vi "4521_Module_configure.vi"() -> ()   [LabVIEW 2010]
panel:
  in  "Port Name":string
  in  "Data Bits":u8=8 min=5 max=8 step=1
  in  "Parity type":bool
  in  "Use parity?":bool
  in  "Stop Bits":bool
  in  "Behaviour":bool
  in  "Enable Checksum?":bool
  in  "422 or 485?":bool
  in  "Append CR?":bool
  in  "485 Baud Rate (9600)":u8(ring)=3 items=["1200 bps", "2400 bps", "4800 bps", "9600 bps", "19.2 kbps", "38.4 kbps"]
  in  "Use checksum":bool
  in  "232 Baud Rate (9600)":u8(ring)=3 items=["1200 bps", "2400 bps", "4800 bps", "9600 bps", "19.2 kbps", "38.4 kbps"]
  out "Reply":string
  out "String Sent":string
  in  "New Address (NN)":u8
  in  "Old Address(AA)":u8
  # "4520 Settings"
  # "Serial Device Settings"
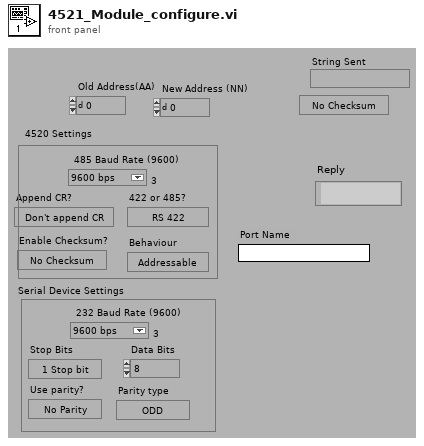
[diagram p1: front panel]
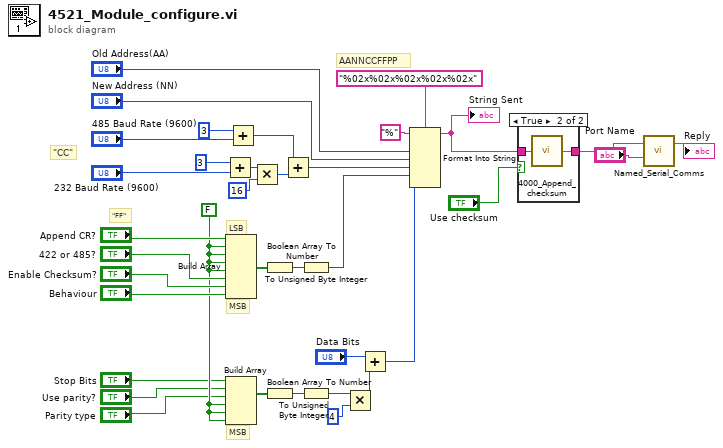
[diagram p0: block diagram]
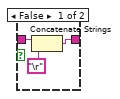
[diagram p2: hidden frame]
diagram:
  w10 = FALSE
  # "\"FF\""
  # "MSB"
  # "AANNCCFFPP"
  # "\"CC\""
  # "MSB"
  # "LSB"
  n1 = Add(x=u8 3, y="232 Baud Rate (9600)") -> (x+y=w22:u8)
  n2 = Build Array("Append CR?", w10, w10, w10, w10, "422 or 485?", "Enable Checksum?", "Behaviour") -> (w32:bool[])
  n3 = Build Array("Stop Bits", "Use parity?", "Parity type", w10, w10, w10) -> (w15:bool[])
  n4 = Add(x=u8 3, y="485 Baud Rate (9600)") -> (x+y=w19:u8)
  n5 = Multiply(x=w22, y=u8 16) -> (x*y=w20:u8)
  n6 = Boolean Array To Number(Boolean array=w32) -> (number=w31:u32)
  n7 = Boolean Array To Number(Boolean array=w15) -> (number=w16:u32)
  n8 = Add(x=w19, y=w20) -> (x+y=w18:u8)
  n9 = To Unsigned Byte Integer(number=w31) -> (unsigned 8bit integer=w17:u8)
  n10 = To Unsigned Byte Integer(number=w16) -> (unsigned 8bit integer=w5:u8)
  n11 = Multiply(x=w5, y=u8 4) -> (x*y=w4:u8)
  n12 = Add(x="Data Bits", y=w4) -> (x+y=w2:u8)
  n13 = Format Into String(format string="%02x%02x%02x%02x%02x", initial string="%", "Old Address(AA)", "New Address (NN)", w18, w17, w2) -> (resulting string=w30:string)  [unwired: 1 in, 1 out]
  "String Sent" <- w30
  n14 = case shown="True" "Use checksum" {
    tunnel: w30 -> [w39 w41]
    tunnel: [w38 w40] -> w26
    frame False {
      n15 = Concatenate Strings(w39, "\r") -> (w38:string)
    }
    frame True {
      n16 = call "4000_Append_checksum.vi"("ADAM command"=w41) -> ("ADAM string to send"=w40:string)
    }
  }
  n17 = call "Named_Serial_Comms.vi"("Write String"=w26, "Port Name"="Port Name") -> ("Read"=→"Reply":string)  [unwired: 10 in, 3 out]
